vi "EXCLUDE_COLOR.vi"() -> (3 "Color Box":u32(colorbox)=13816530)   [LabVIEW 2018, in "CategoryListUIAdapter.lvclass"]
uses:
  CategoryListUIAdapter.lvclass
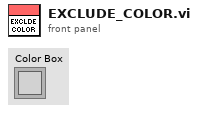
[diagram p1: front panel]
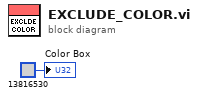
[diagram p0: block diagram]
diagram:
  "Color Box" <- u32 13816530
